vi "5.0.0_Task_Detect_Calibration.vi"(7 "Data in":T1, 8 "error in (no error)":errorcluster, 9 "AllControls In":T2, 10 "?":T3, 11 "Message Queue out":T4) -> (0 "error out":errorcluster, 1 "Flow":string, 2 "Data":T3, 3 "Message Queue Out":T4, 5 "Data out":T1)   [LabVIEW 2017]
uses:
  Depends/AMC/subVIs/TypeDefs/amc_Message Queue.ctl
  Depends/AMC/subVIs/TypeDefs/amc_Message.ctl
  Depends/Tools/Keyed Array/Tools_KeyedArray KeyedArray.ctl
  Ctrls/Data.ctl
  Ctrls/AllControls.ctl
  Ctrls/CSV_Data.ctl
  DIPC 692 Daemon API/typdef/calibration.ctl
  DIPC 692 Daemon API/typdef/task_detect_test_point.ctl
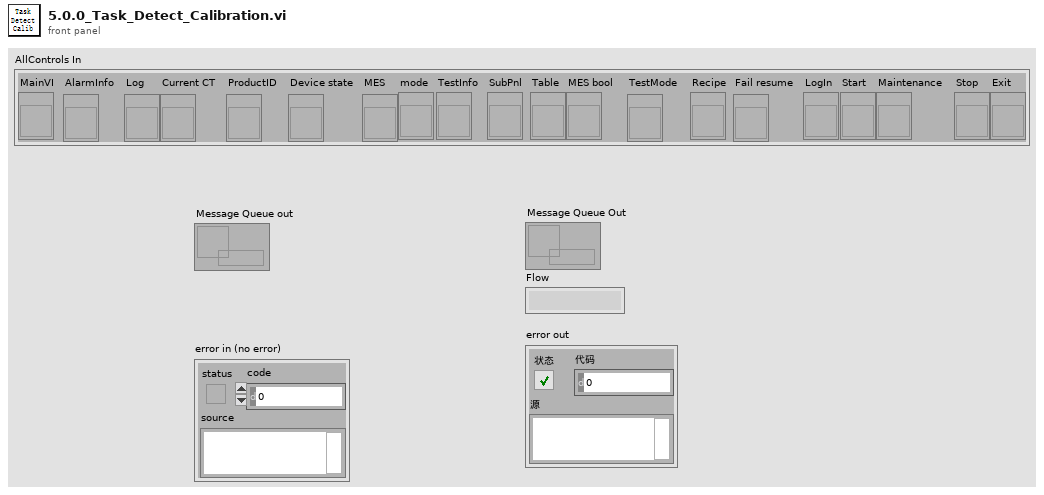
[diagram p1: front panel]
types:
  T1 = typedef "CSV_Data.ctl" = cluster{"Initialisation":cluster{"LMT - Connect UUT (con COM)":string, "LMT - Software Version (rrel)":string, "LMT - Write SKU file (wskuc)":string, "LMT - SKU file name":string, "Connect UUT DDM":string, "Read DDM EOL Timestamp - Mode":string, "Read DDM EOL Timestamp - Timestamp":string, "Read DDM EOL Timestamp - Rig ID":string, "Read DDM EOL Timestamp - Passmark ID":string, "Read DDM EOL Timestamp - Passmark Rev":string, "Software Version before flashing":string, "Read Hardware Serial":string, "UUT DDM SN":string, "Compare DDM SN with MES SN":string, "Backup PCBA Calibration EEPROM Response - CAL":string, "Flash Firmware Version":string, "Check SW Version":string, "Read DDM SW Version after flashing":string, "Set SKU Config":string, "Ready Status":string, "Set Device Mode to EOL":string, "DDM Parameter - Voltage":string, "DDM Parameter - Current":string, "DDM Parameter - Power":string, "DDM Parameter - Speed":string, "DDM Parameter - Pressure":string, "Tester Parameter - Voltage":string, "Tester Parameter - Current":string, "Tester Parameter - Power":string, "Tester Parameter - Ambient Pressure":string, "Tester Parameter - Ambient Temperature":string, "Calculated Parameter - DDM Pressure Corrected":string, "Calculated Parameter - DDM Real Power":string, "Calculated Parameter - Delta V":string}, "BEMF_Calibration":cluster{"Calibration Result - eol_cold_bemf_temp":string, "DDM Ambient Temp":string, "Restriction Plate Diameter":string, "Calibration Result - eol_bemf_mp_cold_coef_a":string, "Calibration Result - eol_bemf_mp_cold_coef_b":string, "Calibration Result - eol_bemf_mp_cold_coef_c":string, "Calibration Result - eol_bemf_lsi_cold_ref_coeffs":string, "Get - Calibration Result - eol_bemf_lsi_speed":string, "Get - Calibration Result - eol_bemf_lsi_integral_0":string, "Calibration Result - eol_bemf_lsi_integral_1":string, "Get - Calibration Result - eol_bemf_lsi_integral_2":string, "Get - Calibration Result - eol_cold_bemf":string, "Get - Calibration Result - eol_cold_bemf_fisf":string, "Finalise Calibration":string, "Compare -Calibration Result - eol_cold_bemf":string, "Compare -Calibration Result - eol_cold_bemf_fisf":string}, "ECO":cluster{"Reset Power Tune":string, "Reset BEMF FISF Calibration":string, "Restriction Plate Diameter":string, "ECO - Stabilisation Time":string, "ECO - DDM Parameter - Voltage":string, "ECO - DDM Parameter - Current":string, "ECO - DDM Parameter - Power":string, "ECO - DDM Parameter - Measured Power":string, "ECO - DDM Parameter - Speed":string, "ECO - DDM Parameter - Pressure":string, "ECO - Tester Parameter - Voltage":string, "ECO - Tester Parameter - Current":string, "ECO - Tester Parameter - Power":string, "ECO - Tester Parameter - Ambient Pressure":string, "ECO - Tester Parameter - Ambient Temperature":string, "ECO - Tester Parameter - Ambient Humidity":string, "ECO - Calculated Parameter - DDM Pressure Corrected":string, "ECO - Calculated Parameter - DDM Real Power":string, "ECO - Calculated Parameter - Delta V":string, "ECO - Calculated Parameter - Flowrate":string, "ECO - Calculated Parameter - Airwatt":string, "ECO - Formula":string, "PT ECO - Power Tune Mode Status":string}, "BOOST":cluster{"Restriction Plate Diameter":string, "BOOST - Stabilisation Time":string, "BOOST - DDM Parameter - Voltage":string, "BOOST - DDM Parameter - Current":string, "BOOST - DDM Parameter - Power":string, "BOOST - DDM Parameter - Measured Power":string, "BOOST - DDM Parameter - Speed":string, "BOOST - DDM Parameter - Pressure":string, "BOOST - Tester Parameter - Voltage":string, "BOOST - Tester Parameter - Current":string, "BOOST - Tester Parameter - Power":string, "BOOST - Tester Parameter - Ambient Pressure":string, "BOOST - Tester Parameter - Ambient Temperature":string, "BOOST - Tester Parameter - Ambient Humidity":string, "BOOST - Calculated Parameter - DDM Pressure Corrected":string, "BOOST - Calculated Parameter - DDM Real Power":string, "BOOST - Calculated Parameter - Delta V":string, "BOOST - Calculated Parameter - Flowrate":string, "BOOST - Calculated Parameter - Airwatt":string, "BOOST - Get AM Presence":string, "Air Muscle Turn Off Status":string, "BOOST - Air Muscle Calculated Parameter - Airwatt B":string, "BOOST - Air Muscle Calculate Airwatt Delta":string, "PT BOOST - Power Tune Mode Status":string, "Finalise Calibration":string, "ECO - Get AW Calibration value":string, "BOOST - Get AW Calibration value":string}, "MAX":cluster{"Restriction Plate Diameter":string, "MAX - Stabilisation Time":string, "Get Average Delta Tmag (LSIdelta_FISFdelta_LSItmag_FISFtmag_IIRtmag)":string, "Get Average Delta Tmag FISF":string, "MAX - DDM Parameter - Voltage":string, "MAX - DDM Parameter - Current":string, "MAX - DDM Parameter - Power":string, "MAX - DDM Parameter - Measured Power":string, "MAX - DDM Parameter - Speed":string, "MAX - DDM Parameter - Pressure":string, "MAX - Tester Parameter - Voltage":string, "MAX - Tester Parameter - Current":string, "MAX - Tester Parameter - Power":string, "MAX - Tester Parameter - Ambient Pressure":string, "MAX - Tester Parameter - Ambient Temperature":string, "MAX - Tester Parameter - Ambient Humidity":string, "MAX - Calculated Parameter - DDM Pressure Corrected":string, "MAX - Calculated Parameter - DDM Real Power":string, "MAX - Calculated Parameter - Delta V":string, "MAX - Calculated Parameter - Flowrate":string, "MAX - Calculated Parameter - Airwatt":string, "MAX_FISF_Check_Average_Delta_Tmag":string, "MAX - FISF - BEMF Finetune Result":string, "MAX tune - Delta P1":string, "MAX tune - Calculated Parameter - Airwatt":string, "Calculate Delta Airwatts - MAX finetune - Delta P2":string, "MAX finetune - DDM Parameter - Voltage":string, "MAX finetune - DDM Parameter - Current":string, "MAX finetune - DDM Parameter - Power":string, "MAX finetune - DDM Parameter - Measured Power":string, "MAX finetune - DDM Parameter - Speed":string, "MAX finetune - DDM Parameter - Pressure":string, "MAX finetune - Tester Parameter - Voltage":string, "MAX finetune - Tester Parameter - Current":string, "MAX finetune - Tester Parameter - Power":string, "MAX finetune - Tester Parameter - Ambient Pressure":string, "MAX finetune - Tester Parameter - Ambient Temperature":string, "MAX finetune - Tester Parameter - Ambient Humidity":string, "MAX finetune - Calculated Parameter - DDM Pressure Corrected":string, "MAX finetune - Calculated Parameter - DDM Real Power":string, "MAX finetune - Calculated Parameter - Delta V":string, "MAX finetune - Calculated Parameter - Flowrate":string, "MAX finetune - Calculated Parameter - Airwatt":string, "Check Derate Result":string, "Delta Tmag FISF":string, "Get Hot BEMF Result":string, "Calculate delta Pressure":string, "Finalise Calibration":string, "Calculate & Check Delta BEMF":string, "Delta P Airwatts Value":string}, "LL":cluster{"DDM Ambient Temp":string, "Restriction Plate Diameter":string, "LL - DDM Parameter - Voltage":string, "LL - DDM Parameter - Current":string, "LL - DDM Parameter - Power":string, "LL - DDM Parameter - Measured Power":string, "LL - DDM Parameter - Speed":string, "LL - DDM Parameter - Pressure":string, "LL - Tester Parameter - Voltage":string, "LL - Tester Parameter - Current":string, "LL - Tester Parameter - Power":string, "LL - DDM Real Power":string, "LL - Calibrate Task Detect LL":string}, "HL":cluster{"HL - DDM Parameter - Voltage":string, "HL - DDM Parameter - Current":string, "HL - DDM Parameter - Power":string, "HL - DDM Parameter - Measured Power":string, "HL - DDM Parameter - Speed":string, "HL - DDM Parameter - Pressure":string, "HL - Tester Parameter - Voltage":string, "HL - Tester Parameter - Current":string, "HL - Tester Parameter - Power":string, "HL - DDM Real Power":string, "HL - Calibrate Task Detect HL":string}, "LH":cluster{"Restriction Plate Diameter":string, "LH - DDM Parameter - Voltage":string, "LH - DDM Parameter - Current":string, "LH - DDM Parameter - Power":string, "LH - DDM Parameter - Measured Power":string, "LH - DDM Parameter - Speed":string, "LH - DDM Parameter - Pressure":string, "LH - Tester Parameter - Voltage":string, "LH - Tester Parameter - Current":string, "LH - Tester Parameter - Power":string, "LH - DDM Real Power":string, "LH - Calibrate Task Detect LH":string}, "HH":cluster{"HH - DDM Parameter - Voltage":string, "HH - DDM Parameter - Current":string, "HH - DDM Parameter - Power":string, "HH - DDM Parameter - Measured Power":string, "HH - DDM Parameter - Speed":string, "HH - DDM Parameter - Pressure":string, "HH - Tester Parameter - Voltage":string, "HH - Tester Parameter - Current":string, "HH - Tester Parameter - Power":string, "HH - DDM Real Power":string, "HH - Calibrate Task Detect HH":string}, "Inlet Blockage Calibration":cluster{"Inlet Blockage Calibration - DDM Parameter - Voltage":string, "Inlet Blockage Calibration - DDM Parameter - Current":string, "Inlet Blockage Calibration - DDM Parameter - Power":string, "Inlet Blockage Calibration - DDM Parameter - Measured Power":string, "Inlet Blockage Calibration - DDM Parameter - Speed":string, "Inlet Blockage Calibration - DDM Parameter - Pressure":string, "Inlet Blockage Calibration - Tester Parameter - Voltage":string, "Inlet Blockage Calibration - Tester Parameter - Current":string, "Inlet Blockage Calibration - Tester Parameter - Power":string, "Inlet Blockage Calibration - DDM Real Power":string, "Calibration Inlet Blockage_E":string, "Finalise Calibration":string, "Get Task Detect LL":string, "Get Task Detect HL":string, "Get Task Detect LH":string, "Get Task Detect HH":string, "Calibration Inlet Blockage":string, "Calibration eol cold bemf temp":string}, "GOOD":cluster{"GOOD UNIT - Clear EEPROM Error Log":string, "GOOD UNIT - Write Product Timestamp - Mode":string, "GOOD UNIT - Write Product Timestamp - Timestamp":string, "GOOD UNIT - Write Product Timestamp - Rig ID":string, "GOOD UNIT - Write Product Timestamp - Passmark ID":string, "GOOD UNIT - Write Product Timestamp - Passmark Rev":string, "GOOD UNIT - Set Device Mode to PROD":string, "GOOD UNIT - Backup PCBA Calibration EEPROM Response":string, "GOOD UNIT - Check Security Bit":string, "GOOD UNIT - Set Calibration Lock":string, "GOOD UNIT - Get_Calibration_Lock":string, "GOOD UNIT - Disconnect UUT":string}, "NG":cluster{"NG UNIT - Read NVM Error":string, "NG UNIT - Set Device Mode to FCT":string, "NG UNIT - Backup PCBA Calibration EEPROM Response - CAL":string, "NG UNIT - Backup PCBA Calibration EEPROM Response - ERROR":string, "NG UNIT - Backup PCBA Calibration EEPROM Response - USAGE":string, "NG UNIT - Disconnect UUT":string}, "SN":string, "Table":string[][], "Count":cluster{"Total":i32, "OK":i32, "NG":i32, "Yield":dbl}, "Start Time":timestamp, "daemon reference":refnum<k5>, "CT":dbl, "Config":string[][], "OK/NG":bool, "Station ID":string, "MES DDM SN":string, "MES PCBA SN":string, "Retest":string, "Lux":string, "Initialisation_Status":cluster{"LMT - Connect UUT (con COM)":string, "LMT - Software Version (rrel)":string, "LMT - Write SKU file (wskuc)":string, "LMT - SKU file name":string, "Connect UUT DDM":string, "Read DDM EOL Timestamp - Mode":string, "Read DDM EOL Timestamp - Timestamp":string, "Read DDM EOL Timestamp - Rig ID":string, "Read DDM EOL Timestamp - Passmark ID":string, "Read DDM EOL Timestamp - Passmark Rev":string, "Software Version before flashing":string, "Read Hardware Serial":string, "UUT DDM SN":string, "Compare DDM SN with MES SN":string, "Backup PCBA Calibration EEPROM Response - CAL":string, "Flash Firmware Version":string, "Check SW Version":string, "Read DDM SW Version after flashing":string, "Set SKU Config":string, "Ready Status":string, "Set Device Mode to EOL":string, "DDM Parameter - Voltage":string, "DDM Parameter - Current":string, "DDM Parameter - Power":string, "DDM Parameter - Speed":string, "DDM Parameter - Pressure":string, "Tester Parameter - Voltage":string, "Tester Parameter - Current":string, "Tester Parameter - Power":string, "Tester Parameter - Ambient Pressure":string, "Tester Parameter - Ambient Temperature":string, "Calculated Parameter - DDM Pressure Corrected":string, "Calculated Parameter - DDM Real Power":string, "Calculated Parameter - Delta V":string}, "BEMF_Calibration_Status":cluster{"Calibration Result - eol_cold_bemf_temp":string, "DDM Ambient Temp":string, "Restriction Plate Diameter":string, "Calibration Result - eol_bemf_mp_cold_coef_a":string, "Calibration Result - eol_bemf_mp_cold_coef_b":string, "Calibration Result - eol_bemf_mp_cold_coef_c":string, "Calibration Result - eol_bemf_lsi_cold_ref_coeffs":string, "Get - Calibration Result - eol_bemf_lsi_speed":string, "Get - Calibration Result - eol_bemf_lsi_integral_0":string, "Calibration Result - eol_bemf_lsi_integral_1":string, "Get - Calibration Result - eol_bemf_lsi_integral_2":string, "Get - Calibration Result - eol_cold_bemf":string, "Get - Calibration Result - eol_cold_bemf_fisf":string, "Finalise Calibration":string, "Compare -Calibration Result - eol_cold_bemf":string, "Compare -Calibration Result - eol_cold_bemf_fisf":string}, "ECO_Status":cluster{"Reset Power Tune":string, "Reset BEMF FISF Calibration":string, "Restriction Plate Diameter":string, "ECO - Stabilisation Time":string, "ECO - DDM Parameter - Voltage":string, "ECO - DDM Parameter - Current":string, "ECO - DDM Parameter - Power":string, "ECO - DDM Parameter - Measured Power":string, "ECO - DDM Parameter - Speed":string, "ECO - DDM Parameter - Pressure":string, "ECO - Tester Parameter - Voltage":string, "ECO - Tester Parameter - Current":string, "ECO - Tester Parameter - Power":string, "ECO - Tester Parameter - Ambient Pressure":string, "ECO - Tester Parameter - Ambient Temperature":string, "ECO - Tester Parameter - Ambient Humidity":string, "ECO - Calculated Parameter - DDM Pressure Corrected":string, "ECO - Calculated Parameter - DDM Real Power":string, "ECO - Calculated Parameter - Delta V":string, "ECO - Calculated Parameter - Flowrate":string, "ECO - Calculated Parameter - Airwatt":string, "ECO - Formula":string, "PT ECO - Power Tune Mode Status":string}, "BOOST_Status":cluster{"Restriction Plate Diameter":string, "BOOST - Stabilisation Time":string, "BOOST - DDM Parameter - Voltage":string, "BOOST - DDM Parameter - Current":string, "BOOST - DDM Parameter - Power":string, "BOOST - DDM Parameter - Measured Power":string, "BOOST - DDM Parameter - Speed":string, "BOOST - DDM Parameter - Pressure":string, "BOOST - Tester Parameter - Voltage":string, "BOOST - Tester Parameter - Current":string, "BOOST - Tester Parameter - Power":string, "BOOST - Tester Parameter - Ambient Pressure":string, "BOOST - Tester Parameter - Ambient Temperature":string, "BOOST - Tester Parameter - Ambient Humidity":string, "BOOST - Calculated Parameter - DDM Pressure Corrected":string, "BOOST - Calculated Parameter - DDM Real Power":string, "BOOST - Calculated Parameter - Delta V":string, "BOOST - Calculated Parameter - Flowrate":string, "BOOST - Calculated Parameter - Airwatt":string, "BOOST - Get AM Presence":string, "Air Muscle Turn Off Status":string, "BOOST - Air Muscle Calculated Parameter - Airwatt B":string, "BOOST - Air Muscle Calculate Airwatt Delta":string, "PT BOOST - Power Tune Mode Status":string, "Finalise Calibration":string, "ECO - Get AW Calibration value":string, "BOOST - Get AW Calibration value":string}, "MAX_Status":cluster{"Restriction Plate Diameter":string, "MAX - Stabilisation Time":string, "Get Average Delta Tmag (LSIdelta_FISFdelta_LSItmag_FISFtmag_IIRtmag)":string, "Get Average Delta Tmag FISF":string, "MAX - DDM Parameter - Voltage":string, "MAX - DDM Parameter - Current":string, "MAX - DDM Parameter - Power":string, "MAX - DDM Parameter - Measured Power":string, "MAX - DDM Parameter - Speed":string, "MAX - DDM Parameter - Pressure":string, "MAX - Tester Parameter - Voltage":string, "MAX - Tester Parameter - Current":string, "MAX - Tester Parameter - Power":string, "MAX - Tester Parameter - Ambient Pressure":string, "MAX - Tester Parameter - Ambient Temperature":string, "MAX - Tester Parameter - Ambient Humidity":string, "MAX - Calculated Parameter - DDM Pressure Corrected":string, "MAX - Calculated Parameter - DDM Real Power":string, "MAX - Calculated Parameter - Delta V":string, "MAX - Calculated Parameter - Flowrate":string, "MAX - Calculated Parameter - Airwatt":string, "MAX_FISF_Check_Average_Delta_Tmag":string, "MAX - FISF - BEMF Finetune Result":string, "MAX tune - Delta P1":string, "MAX tune - Calculated Parameter - Airwatt":string, "Calculate Delta Airwatts - MAX finetune - Delta P2":string, "MAX finetune - DDM Parameter - Voltage":string, "MAX finetune - DDM Parameter - Current":string, "MAX finetune - DDM Parameter - Power":string, "MAX finetune - DDM Parameter - Measured Power":string, "MAX finetune - DDM Parameter - Speed":string, "MAX finetune - DDM Parameter - Pressure":string, "MAX finetune - Tester Parameter - Voltage":string, "MAX finetune - Tester Parameter - Current":string, "MAX finetune - Tester Parameter - Power":string, "MAX finetune - Tester Parameter - Ambient Pressure":string, "MAX finetune - Tester Parameter - Ambient Temperature":string, "MAX finetune - Tester Parameter - Ambient Humidity":string, "MAX finetune - Calculated Parameter - DDM Pressure Corrected":string, "MAX finetune - Calculated Parameter - DDM Real Power":string, "MAX finetune - Calculated Parameter - Delta V":string, "MAX finetune - Calculated Parameter - Flowrate":string, "MAX finetune - Calculated Parameter - Airwatt":string, "Check Derate Result":string, "Delta Tmag FISF":string, "Get Hot BEMF Result":string, "Calculate delta Pressure":string, "Finalise Calibration":string, "Calculate & Check Delta BEMF":string, "Delta P Airwatts Value":string}, "LL_Status":cluster{"DDM Ambient Temp":string, "Restriction Plate Diameter":string, "LL - DDM Parameter - Voltage":string, "LL - DDM Parameter - Current":string, "LL - DDM Parameter - Power":string, "LL - DDM Parameter - Measured Power":string, "LL - DDM Parameter - Speed":string, "LL - DDM Parameter - Pressure":string, "LL - Tester Parameter - Voltage":string, "LL - Tester Parameter - Current":string, "LL - Tester Parameter - Power":string, "LL - DDM Real Power":string, "LL - Calibrate Task Detect LL":string}, "HL_Status":cluster{"HL - DDM Parameter - Voltage":string, "HL - DDM Parameter - Current":string, "HL - DDM Parameter - Power":string, "HL - DDM Parameter - Measured Power":string, "HL - DDM Parameter - Speed":string, "HL - DDM Parameter - Pressure":string, "HL - Tester Parameter - Voltage":string, "HL - Tester Parameter - Current":string, "HL - Tester Parameter - Power":string, "HL - DDM Real Power":string, "HL - Calibrate Task Detect HL":string}, "LH_Status":cluster{"Restriction Plate Diameter":string, "LH - DDM Parameter - Voltage":string, "LH - DDM Parameter - Current":string, "LH - DDM Parameter - Power":string, "LH - DDM Parameter - Measured Power":string, "LH - DDM Parameter - Speed":string, "LH - DDM Parameter - Pressure":string, "LH - Tester Parameter - Voltage":string, "LH - Tester Parameter - Current":string, "LH - Tester Parameter - Power":string, "LH - DDM Real Power":string, "LH - Calibrate Task Detect LH":string}, "HH_Status":cluster{"HH - DDM Parameter - Voltage":string, "HH - DDM Parameter - Current":string, "HH - DDM Parameter - Power":string, "HH - DDM Parameter - Measured Power":string, "HH - DDM Parameter - Speed":string, "HH - DDM Parameter - Pressure":string, "HH - Tester Parameter - Voltage":string, "HH - Tester Parameter - Current":string, "HH - Tester Parameter - Power":string, "HH - DDM Real Power":string, "HH - Calibrate Task Detect HH":string}, "Inlet Blockage Calibration_Status":cluster{"Inlet Blockage Calibration - DDM Parameter - Voltage":string, "Inlet Blockage Calibration - DDM Parameter - Current":string, "Inlet Blockage Calibration - DDM Parameter - Power":string, "Inlet Blockage Calibration - DDM Parameter - Measured Power":string, "Inlet Blockage Calibration - DDM Parameter - Speed":string, "Inlet Blockage Calibration - DDM Parameter - Pressure":string, "Inlet Blockage Calibration - Tester Parameter - Voltage":string, "Inlet Blockage Calibration - Tester Parameter - Current":string, "Inlet Blockage Calibration - Tester Parameter - Power":string, "Inlet Blockage Calibration - DDM Real Power":string, "Calibration Inlet Blockage_E":string, "Finalise Calibration":string, "Get Task Detect LL":string, "Get Task Detect HL":string, "Get Task Detect LH":string, "Get Task Detect HH":string, "Calibration Inlet Blockage":string, "Calibration eol cold bemf temp":string}, "GOOD_Status":cluster{"GOOD UNIT - Clear EEPROM Error Log":string, "GOOD UNIT - Write Product Timestamp - Mode":string, "GOOD UNIT - Write Product Timestamp - Timestamp":string, "GOOD UNIT - Write Product Timestamp - Rig ID":string, "GOOD UNIT - Write Product Timestamp - Passmark ID":string, "GOOD UNIT - Write Product Timestamp - Passmark Rev":string, "GOOD UNIT - Set Device Mode to PROD":string, "GOOD UNIT - Backup PCBA Calibration EEPROM Response":string, "GOOD UNIT - Check Security Bit":string, "GOOD UNIT - Set Calibration Lock":string, "GOOD UNIT - Get_Calibration_Lock":string, "GOOD UNIT - Disconnect UUT":string}, "NG_Status":cluster{"NG UNIT - Read NVM Error":string, "NG UNIT - Set Device Mode to FCT":string, "NG UNIT - Backup PCBA Calibration EEPROM Response - CAL":string, "NG UNIT - Backup PCBA Calibration EEPROM Response - ERROR":string, "NG UNIT - Backup PCBA Calibration EEPROM Response - USAGE":string, "NG UNIT - Disconnect UUT":string}, "SKU":string, "Plate_Diameter":string, "Alarm":string}
  T2 = typedef "AllControls.ctl" = cluster{"MainVI":refnum<vi>, "AlarmInfo":refnum<vi>, "Log":refnum<vi>, "Current CT":refnum<vi>, "ProductID":refnum<vi>, "Device state":refnum<vi>, "MES":refnum<vi>, "mode":refnum<vi>, "TestInfo":refnum<vi>, "SubPnl":refnum<vi>, "Table":refnum<vi>, "MES bool":refnum<vi>, "TestMode":refnum<vi>, "Recipe":refnum<vi>, "Fail resume":refnum<vi>, "LogIn":refnum<vi>, "Start":refnum<vi>, "Maintenance":refnum<vi>, "Stop":refnum<vi>, "Exit":refnum<vi>}
  T3 = typedef "Data.ctl" = cluster{"Initialisation":cluster{"DDM_Parameter":dbl[], "DDM_Parameter_status":bool[], "Get_Tester_Parameter":dbl[], "Get_Tester_Parameter_status":bool[], "Cal_Tester_Parameter":dbl[], "Cal_Tester_Parameter_status":bool[], "sw_version_before_status":bool, "sw_version_after_status":bool, "Set_SKU_Config_With_LMT_status":bool, "FCT_timestamp_status":bool, "LMT_Connect_to_UUT_status":bool}, "BEMF_Calibration":cluster{"Read_ambient_temperature":dbl, "Calibration_Vaule":dbl[], "Calibration_Vaule _B":dbl[], "Calibration_Vaule_status":bool[], "Calibration_Vaule_B_status":bool[]}, "ECO":cluster{"DDM_Parameter":dbl[], "DDM_Parameter_status":bool[], "Get_Tester_Parameter":dbl[], "Get_Tester_Parameter_status":bool[], "Cal_Tester_Parameter":dbl[], "Cal_Tester_Parameter_status":bool[], "DDM_Parameter_after_power_tune":dbl[], "Get_Tester_Parameter_after_power_tune":dbl[], "Cal_Tester_Parameter_after_power_tune":dbl[], "Cal_Tester_Parameter_after_power_tune_status":bool[], "Delta_P":dbl}, "BOOST":cluster{"DDM_Parameter":dbl[], "DDM_Parameter_status":bool[], "Get_Tester_Parameter":dbl[], "Get_Tester_Parameter_status":bool[], "Cal_Tester_Parameter":dbl[], "Cal_Tester_Parameter_status":bool[], "DDM_Parameter_after_power_tune":dbl[], "Get_Tester_Parameter_after_power_tune":dbl[], "Cal_Tester_Parameter_after_power_tune":dbl[], "Cal_Tester_Parameter_after_power_tune_status":bool[], "airwatts_am_off":dbl, "AW_Delta_(AM_on_and_off)":dbl, "AW_Delta_(AM_on_and_off)_Status":bool, "Delta_P":dbl}, "MAX":cluster{"Average_Tmag_Data":cluster{"LSI Delta in degC":dbl, "FISF Delta in degc":dbl, "LSI Tmag in degC":dbl, "Fisf Tmag in degC":dbl, "IIR Tmag in degC":dbl}, "DDM_Parameter":dbl[], "DDM_Parameter_status":bool[], "Get_Tester_Parameter":dbl[], "Get_Tester_Parameter_status":bool[], "Cal_Tester_Parameter":dbl[], "BEMF_Finetune":cluster{"eol_bemf_mp_cold_coef_c":dbl, "eol_cold_bemf_fisf_offset":dbl}, "AW_Tune":cluster{"delta_P1":dbl, "delta_P_Setting":dbl}, "DDM_Parameter_after_Airwatts_Tune":dbl[], "Get_Tester_Parameter_after_Airwatts_Tune":dbl[], "Cal_Tester_Parameter_after_Airwatts_Tune":dbl[], "DDM_Parameter_after_Airwatts_Finetune":dbl[], "Get_Tester_Parameter_after_Airwatts_Finetune":dbl[], "Cal_Tester_Parameter_after_Airwatts_Finetune":dbl[], "AW_Finetune":cluster{"delta_P2":dbl, "delta_P_Setting":dbl}, "Delta_Tmag_after_tune":cluster{"LSI Delta in degC":dbl, "FISF Delta in degc":dbl, "LSI Tmag in degC":dbl, "Fisf Tmag in degC":dbl, "IIR Tmag in degC":dbl}, "Hot Bemf in mV":dbl, "DDM_Pressure":dbl, "Delta_Pressure":dbl, " Cold Bemf in mV":dbl, " delta Bemf":dbl, " delta p":dbl, "Delta_Pressure_status":bool, " delta Bemf_status":bool, "LSI Delta in degC_status":bool, "FISF Delta in degc_status":bool, "Max_check_derate_status_status":bool, "Average_All_data":dbl[][], "Average_Tmag_Data_status":bool[], "Average_Tmag_Data_after_tune_status":bool[], "Cal_Tester_Parameter_status":bool[], "Cal_Tester_Parameter_status_after_Airwatts_Tune":bool[], "Cal_Tester_Parameter_status_after_Airwatts_FineTune":bool[]}, "Task_Detect_Calib":cluster{"LL":cluster{"DDM_Parameter":dbl[], "DDM_Parameter_status":bool[], "Get_Tester_Parameter":dbl[], "Get_Tester_Parameter_status":bool[], "Set_task_detect_A":dbl, "Set_task_detect_A_Status":bool}, "HL":cluster{"DDM_Parameter":dbl[], "DDM_Parameter_status":bool[], "Get_Tester_Parameter":dbl[], "Get_Tester_Parameter_status":bool[], "Set_task_detect_B":dbl, "Set_task_detect_B_Status":bool}, "LH":cluster{"DDM_Parameter":dbl[], "DDM_Parameter_status":bool[], "Get_Tester_Parameter":dbl[], "Get_Tester_Parameter_status":bool[], "Set_task_detect_C":dbl, "Set_task_detect_C_Status":bool}, "HH":cluster{"DDM_Parameter":dbl[], "DDM_Parameter_status":bool[], "Get_Tester_Parameter":dbl[], "Get_Tester_Parameter_status":bool[], "Set_task_detect_D":dbl, "Read_and_check_calibration_Status":bool[], "Set_task_detect_D_Status":bool}, "Get_eol_inlet_blockage_E":dbl, "Calib_vaule":cluster{"Get_task_detect_LL":dbl, "Get_task_detect_HL":dbl, "Get_task_detect_LH":dbl, "Get_task_detect_HH":dbl, "eol_inlet_blockage":dbl, "eol_code_bemf_temp":dbl}, "calibrated temp":dbl, "Inlet_Blockage_Calibration":cluster{"DDM_Parameter":dbl[], "DDM_Parameter_status":bool[], "Get_Tester_Parameter":dbl[], "Get_Tester_Parameter_status":bool[]}, "Get_eol_inlet_blockage_E_Status":bool}, "good":cluster{"Write_Product_TS":cluster{"TIMESTAMP":i64, "RIG_ID":i64, "PASSMARK_ID":i64, "PASSMARK_REV":i64}, "Read_Product_TS":cluster{"TIMESTAMP":i64, "RIG_ID":i64, "PASSMARK_ID":i64, "PASSMARK_REV":i64}, "Good_Check_Secuity_Bit_Stauts":bool}}
  T4 = typedef "amc_Message Queue.ctl" = refnum<queue>
  T5 = typedef "HD Config.ctl" = cluster{" PC":cluster{"PC Address":u8[], "PC Port":i32}, "FCO":cluster{"COM":refnum<visa-resource-name>, "Baudrate":u32}, "DC Power ":cluster{"COM":refnum<visa-resource-name>, "Baudrate":u32}, "PW3336":cluster{"COM":refnum<visa-resource-name>, "Baudrate":u32}, "Lefoo":cluster{"COM":refnum<visa-resource-name>, "Baudrate":u32}, "Tempt&Hum":cluster{"COM":refnum<visa-resource-name>, "Baudrate":u32}, "DIPC":cluster{"COM":refnum<visa-resource-name>}, "Daemon":cluster{"IP Address":string, "Port":u16, "Retry":u16}, "URAT":cluster{"COM":refnum<visa-resource-name>, "Baudrate":u32}, "Fail_resume_mode":bool, "GRR":bool}
  T6 = typedef "calibration.ctl" = string
  T7 = typedef "task_detect_test_point.ctl" = enum16{"LL", "HL", "LH", "HH"}
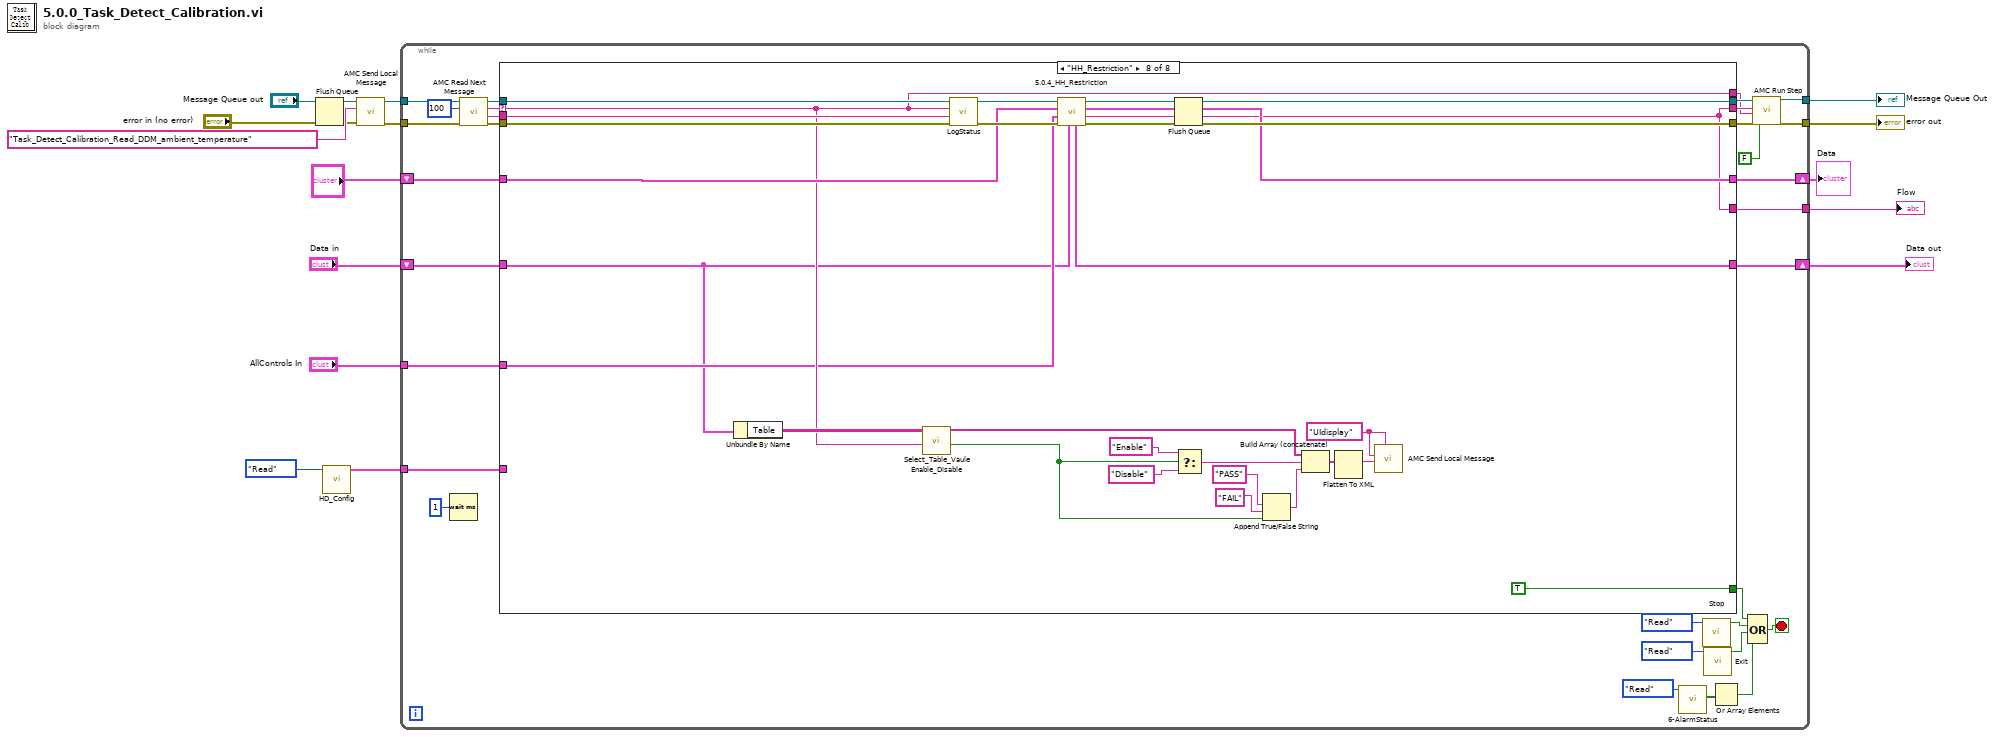
[diagram p0: block diagram]
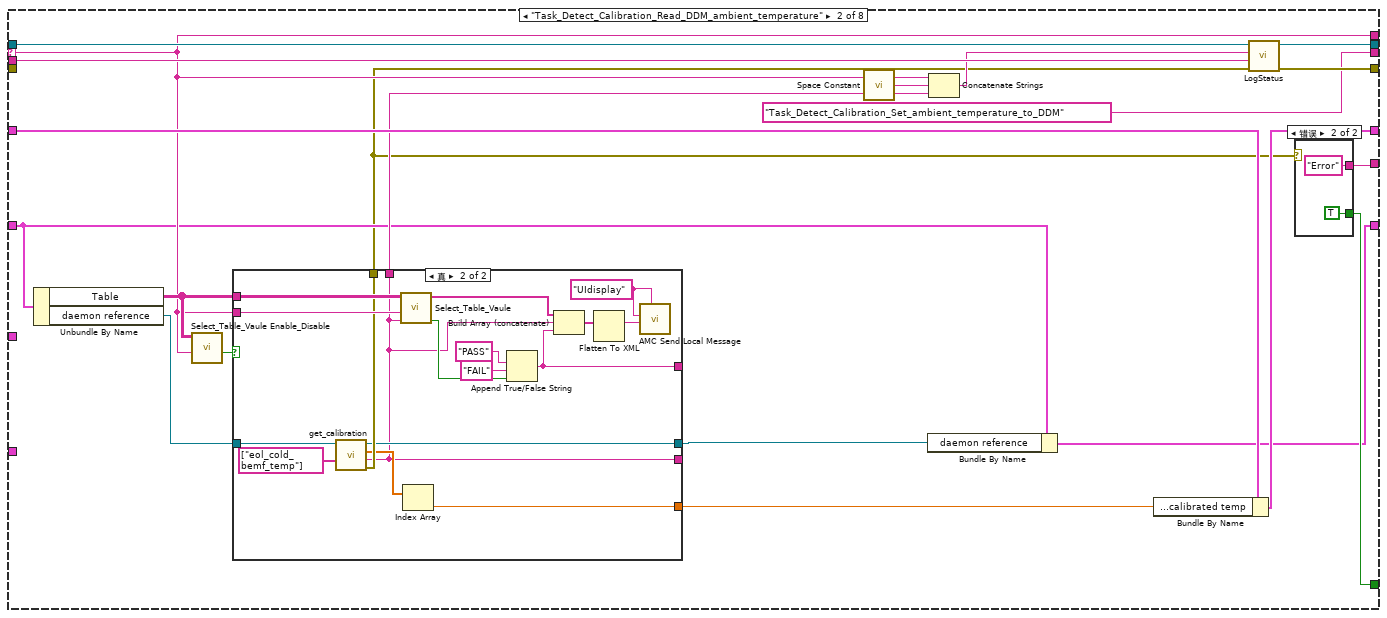
[diagram p3: hidden frame]
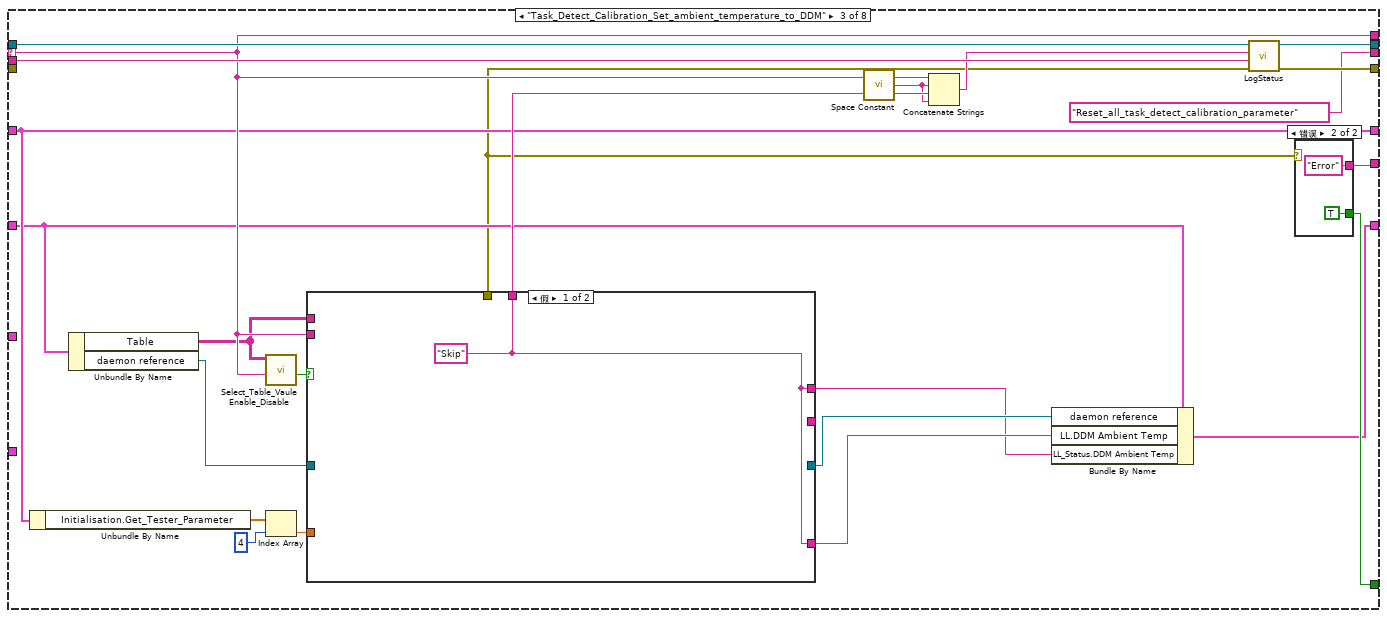
[diagram p6: hidden frame]
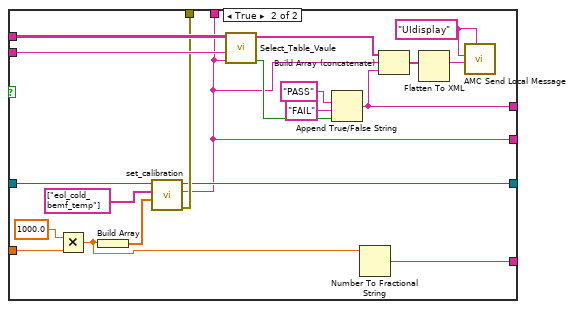
[diagram p8: hidden frame]
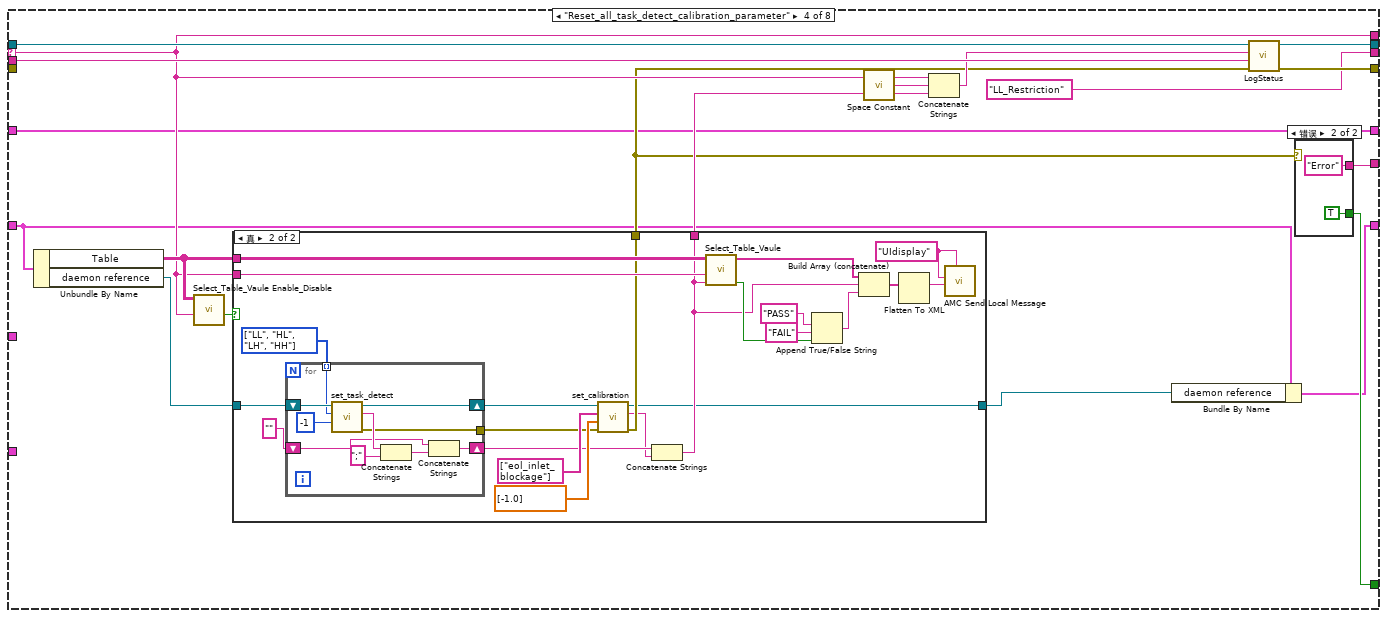
[diagram p9: hidden frame]
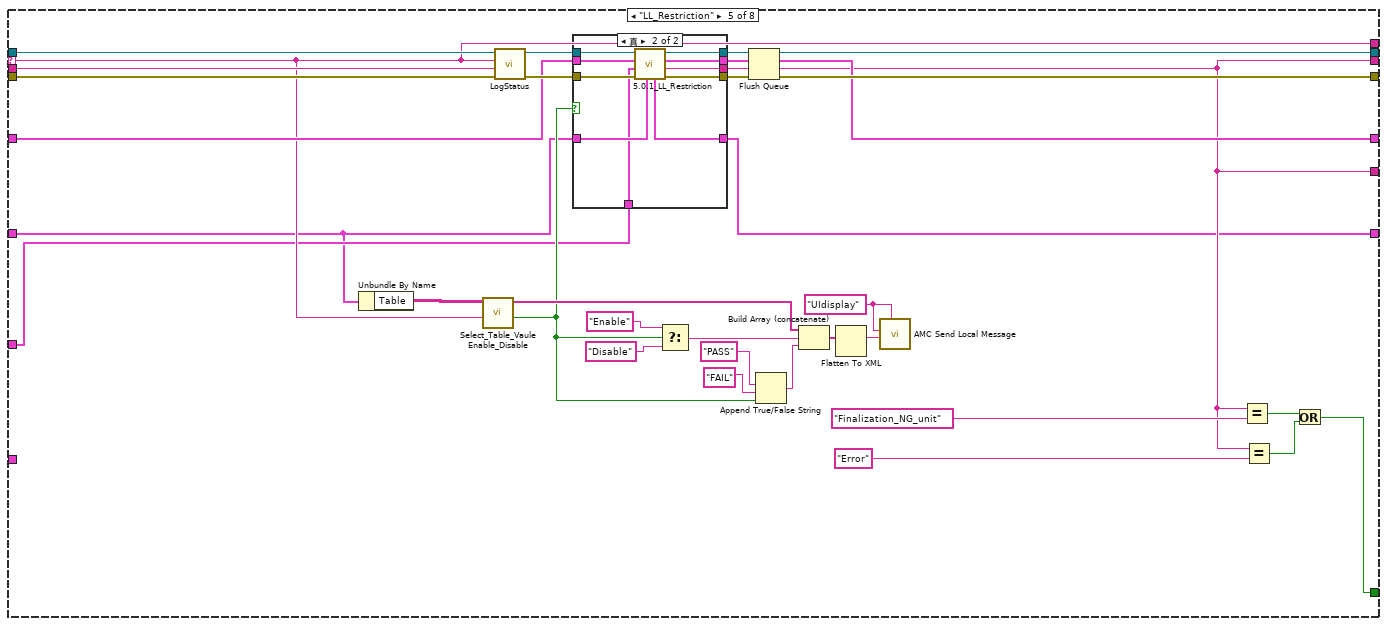
[diagram p12: hidden frame]
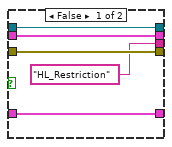
[diagram p13: hidden frame]
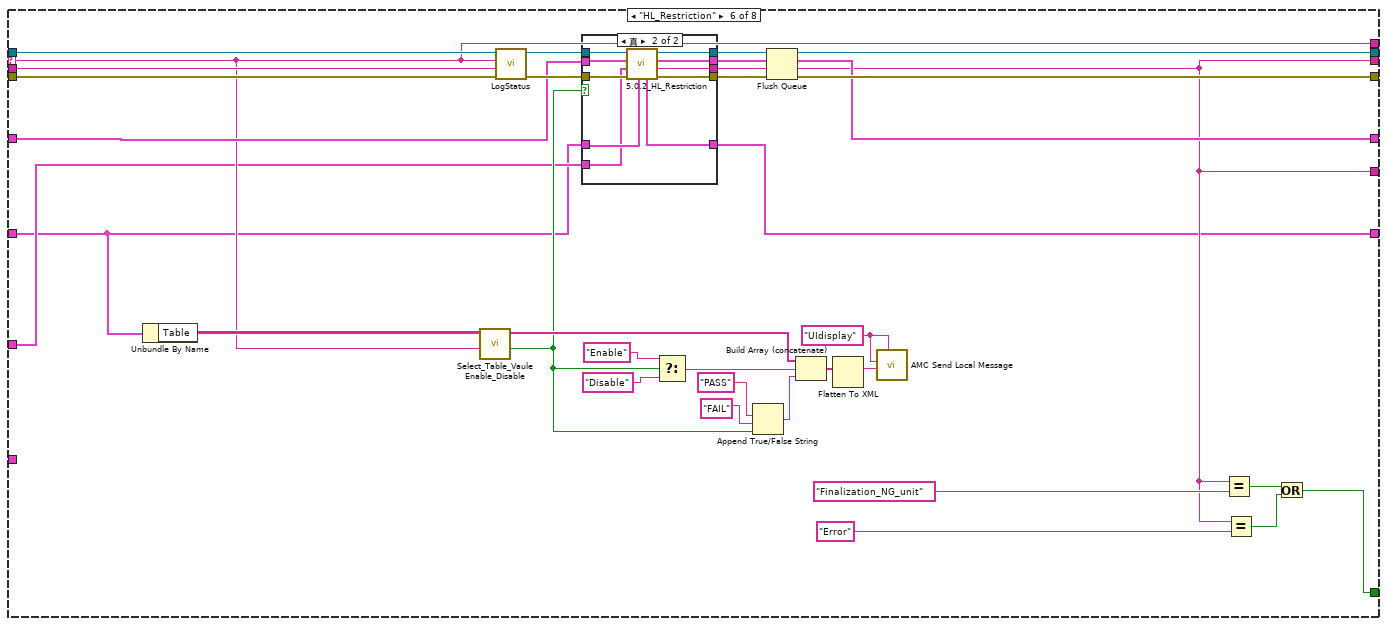
[diagram p14: hidden frame]
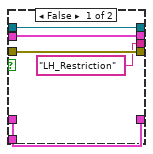
[diagram p15: hidden frame]
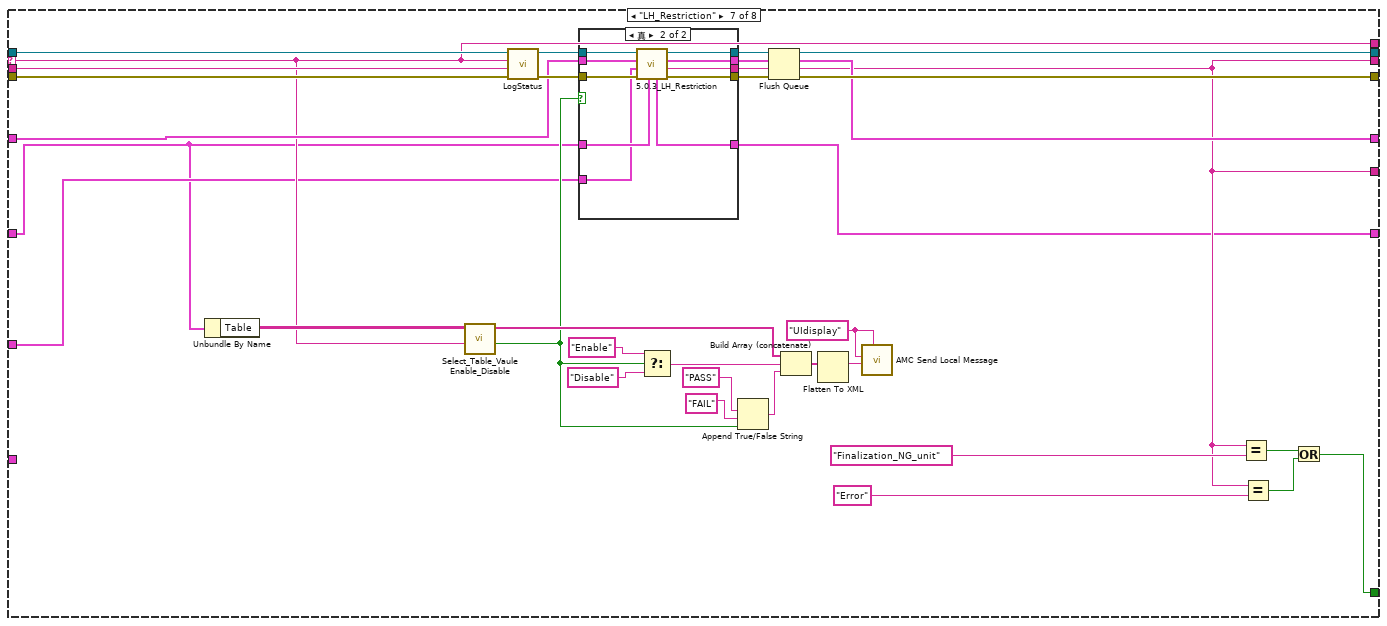
[diagram p16: hidden frame]
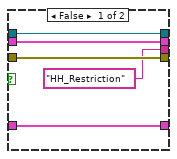
[diagram p17: hidden frame]
diagram:
  n1 = Flush Queue(queue="Message Queue out") -> (queue out=w4:T4)  [unwired: 1 in, 2 out]
  n2 = call "HD_Config.vi"("Step"=enum16{"Initial", "Write", "Read"}."Read") -> ("HD Config out"=w8:T5)  [unwired: 9 in, 1 out]
  n3 = call "AMC Send Local Message.vi"("error in (no error)"="error in (no error)", "Message Name"="Task_Detect_Calibration_Read_DDM_ambient_temperature", "Message Queue in"=w4) -> ("error out"=w13:errorcluster, "Message Queue out"=w14:T4)  [unwired: 7 in]
  n4 = while {
    tunnel: w14 -> [w47]
    tunnel: [w43] -> w6
    tunnel: w13 -> [w41]
    tunnel: [w38] -> w5
    shift-right: [w34] -> w10
    shift-left: "?" -> [w35]
    tunnel: w8 -> [w33]
    tunnel: [w29] -> w7
    shift-right: [w21] -> w2
    shift-left: "Data in" -> [w22]
    tunnel: "AllControls In" -> [w20]
    stop <- w23 stop-if-true
    n5 = Wait (ms)(milliseconds to wait=u32 1 ("等待时间（毫秒）")) -> ()  [unwired: 1 out]
    n6 = call "AMC Read Next Message.vi"("error in (no error)"=w41, "timeout (1ms)"=100, "Message Queue in"=w47) -> ("error out"=w40:errorcluster, "Message Value"=w31:string, "Message Name"=w45:string, "Message Queue out"=w46:T4)  [unwired: 1 in, 4 out]
    n7 = case shown="\"HH_Restriction\"" w45 {
      selector: w45 -> [_ w62 w108 w147 w197 w241 w287 w333]
      tunnel: w46 -> [w51 w71 w114 w155 w217 w263 w309 w351]
      tunnel: [w51 w71 w114 w155 w201 w253 w299 w345] -> w44
      tunnel: w40 -> [w50 _ _ _ w221 w267 w313 w355]
      tunnel: [w50 w70 w113 w154 w218 w264 w310 w352] -> w39
      tunnel: [_ w58 w105 w143 w206 w254 w301 TRUE] -> w24
      tunnel: w35 -> [w49 w67 w99 w141 w208 w260 w306 w348]
      tunnel: [w49 w56 w99 w141 w215 w261 w307 w349] -> w34
      tunnel: w31 -> [_ w69 w112 w153 w220 w266 w312 w354]
      tunnel: [_ w62 w108 w147 w197 w241 w287 w333] -> w30
      tunnel: w33 -> [_ _ _ _ _ _ _ _]
      tunnel: [_ "Task_Detect_Calibration_Set_ambient_temperature_to_DDM" "Reset_all_task_detect_calibration_parameter" "LL_Restriction" w202 w255 w300 w347] -> w32
      tunnel: [_ w59 w106 w144 w202 w255 w300 w347] -> w29
      tunnel: w22 -> [w48 w55 w98 w140 w191 w237 w283 w329]
      tunnel: [w48 w53 w97 w139 w193 w239 w285 w330] -> w21
      tunnel: w20 -> [_ _ _ _ w192 w238 w284 w331]
      frame "假", Default {
      }
      frame "Task_Detect_Calibration_Read_DDM_ambient_temperature" {
        n8 = Unbundle By Name(w55) -> ("Table"=w63:string[][], "daemon reference"=w60:refnum<k5>)
        n9 = call "Select_Table_Vaule Enable_Disable.vi"("Action"=w62, "Table"=w63) -> ("Enable"=w61:bool)  [unwired: 8 in, 1 out]
        n10 = case shown="真" w61 {
          tunnel: [_ w76] -> w64
          tunnel: w63 -> [_ w84]
          tunnel: w62 -> [_ w83]
          tunnel: w60 -> [w74 w81]
          tunnel: [_ w80] -> w54
          tunnel: [w74 w78] -> w52
          tunnel: [_ w77] -> w57
          tunnel: [_ w76] -> _
          tunnel: [_ w75] -> _
          frame False {
          }
          frame True {
            w90 = "UIdisplay" ("Process (\"\" - local)")
            n11 = call "get_calibration.vi"("Calibration"=T6[] ["eol_cold_bemf_temp"], "daemon reference in"=w81) -> ("error out"=w80:errorcluster, "response"=w76:string, "values"=w79:dbl[], "daemon reference out"=w78:refnum<k5>)  [unwired: 5 in, 1 out]
            n12 = call "Select_Table_Vaule.vi"("Vaule"=w76, "Action"=w83, "Table"=w84) -> ("Result"=w85:bool, "vaule"=w91:string[])  [unwired: 7 in]
            n13 = Index Array(array=w79) -> (element=w77:dbl)  [unwired: 1 in]
            n14 = Append True/False String(1:w85, 2:"FAIL" ("真字符串"), 3:"PASS" ("真字符串")) -> (0:w75:string)  [unwired: 1 in]
            n15 = Build Array (concatenate)(w91, w76, w75) -> (w89:string[])
            n16 = Flatten To XML(anything=w89) -> (xml string=w88:string)
            n17 = call "AMC Send Local Message.vi"("Process (\"\" - local)"=w90, "Message Value"=w88, "Message Name"=w90) -> ()  [unwired: 7 in, 2 out]
          }
        }
        n18 = call <vilib>:"Space Constant.vi"() -> ("String"=w65:string)
        n19 = Bundle By Name(cluster=w55, "daemon reference"=w52) -> (w53:T1)
        n20 = Concatenate Strings(w62, w65, w64) -> (w66:string)
        n21 = Bundle By Name(cluster=w67, "Task_Detect_Calib.calibrated temp"=w57) -> (w56:T3)
        n22 = call "LogStatus.vi"("error in (no error)"=w54, "last message"=w69, "message"=w66) -> ("error  out"=w70:errorcluster)  [unwired: 8 in]
        n23 = case shown="错误" w54 {
          tunnel: [_ TRUE] -> w58
          tunnel: [_ "Error"] -> w59
          frame No Error {
          }
          frame Error {
          }
        }
      }
      frame "Task_Detect_Calibration_Set_ambient_temperature_to_DDM" {
        n24 = Unbundle By Name(w99) -> ("Initialisation.Get_Tester_Parameter"=w104:dbl[])
        n25 = Unbundle By Name(w98) -> ("Table"=w101:string[][], "daemon reference"=w100:refnum<k5>)
        n26 = call "Select_Table_Vaule Enable_Disable.vi"("Action"=w108, "Table"=w101) -> ("Enable"=w107:bool)  [unwired: 8 in, 1 out]
        n27 = Index Array(array=w104, index=4) -> (element=w103:dbl)
        n28 = case shown="假" w107 {
          tunnel: [w117 w121] -> w109
          tunnel: w101 -> [_ w130]
          tunnel: w108 -> [_ w129]
          tunnel: w100 -> [_ w126]
          tunnel: [_ w127] -> w95
          tunnel: w103 -> [_ w125]
          tunnel: [_ w122] -> w96
          tunnel: [_ w121] -> _
          tunnel: [w117 w120] -> w92
          tunnel: [w117 w118] -> w93
          frame False {
            w117 = "Skip" ("response")
          }
          frame True {
            w136 = "UIdisplay" ("Process (\"\" - local)")
            n29 = Multiply(x=1000.0, y=w125) -> (x*y=w119:dbl)
            n30 = Build Array(w119) -> (w124:dbl[])
            n31 = call "set_calibration.vi"("values"=w124, "calibration"=T6[] ["eol_cold_bemf_temp"], "daemon reference in"=w126) -> ("error out"=w127:errorcluster, "response"=w121:string, "daemon reference out"=w122:refnum<k5>)  [unwired: 5 in, 1 out]
            n32 = call "Select_Table_Vaule.vi"("Vaule"=w121, "Action"=w129, "Table"=w130) -> ("Result"=w131:bool, "vaule"=w137:string[])  [unwired: 7 in]
            n33 = Append True/False String(1:w131, 2:"FAIL" ("真字符串"), 3:"PASS" ("真字符串")) -> (0:w120:string)  [unwired: 1 in]
            n34 = Number To Fractional String(number=w119) -> (F-format string=w118:string)  [unwired: 3 in]
            n35 = Build Array (concatenate)(w137, w121, w120) -> (w135:string[])
            n36 = Flatten To XML(anything=w135) -> (xml string=w134:string)
            n37 = call "AMC Send Local Message.vi"("Process (\"\" - local)"=w136, "Message Value"=w134, "Message Name"=w136) -> ()  [unwired: 7 in, 2 out]
          }
        }
        n38 = call <vilib>:"Space Constant.vi"() -> ("String"=w94:string)
        n39 = Concatenate Strings(w108, w94, w109, w94) -> (w110:string)
        n40 = Bundle By Name(cluster=w98, "daemon reference"=w96, "LL.DDM Ambient Temp"=w93, "LL_Status.DDM Ambient Temp"=w92) -> (w97:T1)
        n41 = call "LogStatus.vi"("error in (no error)"=w95, "last message"=w112, "message"=w110) -> ("error  out"=w113:errorcluster)  [unwired: 8 in]
        n42 = case shown="错误" w95 {
          tunnel: [_ TRUE] -> w105
          tunnel: [_ "Error"] -> w106
          frame No Error {
          }
          frame Error {
          }
        }
      }
      frame "Reset_all_task_detect_calibration_parameter" {
        n43 = Unbundle By Name(w140) -> ("Table"=w148:string[][], "daemon reference"=w145:refnum<k5>)
        n44 = call "Select_Table_Vaule Enable_Disable.vi"("Action"=w147, "Table"=w148) -> ("Enable"=w146:bool)  [unwired: 8 in, 1 out]
        n45 = case shown="真" w146 {
          tunnel: [_ w163] -> w149
          tunnel: w148 -> [_ w172]
          tunnel: w147 -> [_ w171]
          tunnel: w145 -> [w158 w170]
          tunnel: [_ w161] -> w142
          tunnel: [w158 w159] -> w138
          frame False {
          }
          frame True {
            w167 = T7[] [enum."LL", enum."HL", enum."LH", enum."HH"] items=["LL", "HL", "LH", "HH"]
            w179 = "UIdisplay" ("Process (\"\" - local)")
            n46 = for {
              tunnel: w167 -> [w187] mode=indexing
              shift-right: [w189] -> w165
              shift-left: w170 -> [w190]
              shift-right: [w184] -> w164
              shift-left: "" -> [w183]
              tunnel: [w181] -> w162
              n47 = call "set_task_detect.vi"("Action"=-1, "Test Point"=w187, "daemon reference in"=w190) -> ("error out"=w181:errorcluster, "response"=w188:string, "daemon reference out"=w189:refnum<k5>)  [unwired: 5 in, 1 out]
              n48 = Concatenate Strings(w188, ";" ("字符串")) -> (w182:string)
              n49 = Concatenate Strings(w183, w182) -> (w184:string)
            }
            n50 = call "set_calibration.vi"("error in (no error)"=w162, "values"=dbl[] [-1.0], "calibration"=T6[] ["eol_inlet_blockage"], "daemon reference in"=w165) -> ("error out"=w161:errorcluster, "response"=w160:string, "daemon reference out"=w159:refnum<k5>)  [unwired: 4 in, 1 out]
            n51 = Concatenate Strings(w164, w160) -> (w163:string)
            n52 = call "Select_Table_Vaule.vi"("Vaule"=w163, "Action"=w171, "Table"=w172) -> ("Result"=w173:bool, "vaule"=w180:string[])  [unwired: 7 in]
            n53 = Append True/False String(1:w173, 2:"FAIL" ("真字符串"), 3:"PASS" ("真字符串")) -> (0:w174:string)  [unwired: 1 in]
            n54 = Build Array (concatenate)(w180, w163, w174) -> (w178:string[])
            n55 = Flatten To XML(anything=w178) -> (xml string=w177:string)
            n56 = call "AMC Send Local Message.vi"("Process (\"\" - local)"=w179, "Message Value"=w177, "Message Name"=w179) -> ()  [unwired: 7 in, 2 out]
          }
        }
        n57 = call <vilib>:"Space Constant.vi"() -> ("String"=w150:string)
        n58 = Concatenate Strings(w147, w150, w149) -> (w151:string)
        n59 = Bundle By Name(cluster=w140, "daemon reference"=w138) -> (w139:T1)
        n60 = call "LogStatus.vi"("error in (no error)"=w142, "last message"=w153, "message"=w151) -> ("error  out"=w154:errorcluster)  [unwired: 8 in]
        n61 = case shown="错误" w142 {
          tunnel: [_ TRUE] -> w143
          tunnel: [_ "Error"] -> w144
          frame No Error {
          }
          frame Error {
          }
        }
      }
      frame "LL_Restriction" {
        w209 = "UIdisplay" ("Process (\"\" - local)")
        n62 = Unbundle By Name(w191) -> ("Table"=w198:string[][])
        n63 = call "Select_Table_Vaule Enable_Disable.vi"("Action"=w197, "Table"=w198) -> ("Enable"=w195:bool, "vaule"=w196:string[])  [unwired: 8 in]
        n64 = call "LogStatus.vi"("error in (no error)"=w221, "last message"=w220, "message"=w197) -> ("error  out"=w219:errorcluster)  [unwired: 8 in]
        n65 = case shown="真" w195 {
          tunnel: w219 -> [w224 w236]
          tunnel: [w224 w235] -> w218
          tunnel: w217 -> [w226 w234]
          tunnel: [w226 w233] -> w216
          tunnel: [w225 w232] -> w215
          tunnel: w208 -> [w225 w231]
          tunnel: ["HL_Restriction" w230] -> w202
          tunnel: w191 -> [w222 w229]
          tunnel: [w222 w228] -> w193
          tunnel: w192 -> [_ w227]
          frame False {
          }
          frame True {
            n66 = call "5.0.1_LL_Restriction.vi"("Data in"=w229, "error in (no error)"=w236, "AllControls In"=w227, 10:w231, "Message Queue out"=w234) -> ("error out"=w235:errorcluster, "Flow"=w230:string, "Data"=w232:T3, "Message Queue Out"=w233:T4, "Data out"=w228:T1)  [unwired: 2 in]
          }
        }
        n67 = Select(t="Enable" ("元素"), s=w195, f="Disable" ("元素")) -> (s? t:f=w194:string)
        n68 = Flush Queue(queue=w216) -> (queue out=w201:T4)  [unwired: 1 in, 2 out]
        n69 = Append True/False String(1:w195, 2:"FAIL" ("真字符串"), 3:"PASS" ("真字符串")) -> (0:w214:string)  [unwired: 1 in]
        n70 = Build Array (concatenate)(w196, w194, w214) -> (w212:string[])
        n71 = Flatten To XML(anything=w212) -> (xml string=w213:string)
        n72 = call "AMC Send Local Message.vi"("Process (\"\" - local)"=w209, "Message Value"=w213, "Message Name"=w209) -> ()  [unwired: 7 in, 2 out]
        n73 = Equal?(x=w202, y="Finalization_NG_unit") -> (x = y?=w205:bool)
        n74 = Equal?(x=w202, y="Error") -> (x = y?=w203:bool)
        n75 = Or(x=w205, y=w203) -> (x .or. y?=w206:bool)
      }
      frame "HL_Restriction" {
        w247 = "UIdisplay" ("Process (\"\" - local)")
        n76 = Unbundle By Name(w237) -> ("Table"=w242:string[][])
        n77 = call "Select_Table_Vaule Enable_Disable.vi"("Action"=w241, "Table"=w242) -> ("Enable"=w240:bool, "vaule"=w244:string[])  [unwired: 8 in]
        n78 = call "LogStatus.vi"("error in (no error)"=w267, "last message"=w266, "message"=w241) -> ("error  out"=w265:errorcluster)  [unwired: 8 in]
        n79 = case shown="真" w240 {
          tunnel: w265 -> [w270 w282]
          tunnel: [w270 w281] -> w264
          tunnel: w263 -> [w272 w280]
          tunnel: [w272 w279] -> w262
          tunnel: [w271 w278] -> w261
          tunnel: w260 -> [w271 w277]
          tunnel: ["LH_Restriction" w276] -> w255
          tunnel: w237 -> [w268 w275]
          tunnel: [w268 w274] -> w239
          tunnel: w238 -> [_ w273]
          frame False {
          }
          frame True {
            n80 = call "5.0.2_HL_Restriction.vi"("Data in"=w275, "error in (no error)"=w282, "AllControls In"=w273, 10:w277, "Message Queue out"=w280) -> ("error out"=w281:errorcluster, "Flow"=w276:string, "Data"=w278:T3, "Message Queue Out"=w279:T4, "Data out"=w274:T1)  [unwired: 2 in]
          }
        }
        n81 = Select(t="Enable" ("元素"), s=w240, f="Disable" ("元素")) -> (s? t:f=w243:string)
        n82 = Append True/False String(1:w240, 2:"FAIL" ("真字符串"), 3:"PASS" ("真字符串")) -> (0:w252:string)  [unwired: 1 in]
        n83 = Flush Queue(queue=w262) -> (queue out=w253:T4)  [unwired: 1 in, 2 out]
        n84 = Build Array (concatenate)(w244, w243, w252) -> (w250:string[])
        n85 = Flatten To XML(anything=w250) -> (xml string=w251:string)
        n86 = call "AMC Send Local Message.vi"("Process (\"\" - local)"=w247, "Message Value"=w251, "Message Name"=w247) -> ()  [unwired: 7 in, 2 out]
        n87 = Equal?(x=w255, y="Finalization_NG_unit") -> (x = y?=w258:bool)
        n88 = Equal?(x=w255, y="Error") -> (x = y?=w256:bool)
        n89 = Or(x=w258, y=w256) -> (x .or. y?=w254:bool)
      }
      frame "LH_Restriction" {
        w293 = "UIdisplay" ("Process (\"\" - local)")
        n90 = Unbundle By Name(w283) -> ("Table"=w288:string[][])
        n91 = call "Select_Table_Vaule Enable_Disable.vi"("Action"=w287, "Table"=w288) -> ("Enable"=w286:bool, "vaule"=w290:string[])  [unwired: 8 in]
        n92 = call "LogStatus.vi"("error in (no error)"=w313, "last message"=w312, "message"=w287) -> ("error  out"=w311:errorcluster)  [unwired: 8 in]
        n93 = case shown="真" w286 {
          tunnel: w311 -> [w316 w328]
          tunnel: [w316 w327] -> w310
          tunnel: w309 -> [w318 w326]
          tunnel: [w318 w325] -> w308
          tunnel: [w317 w324] -> w307
          tunnel: w306 -> [w317 w323]
          tunnel: ["HH_Restriction" w322] -> w300
          tunnel: [w314 w320] -> w285
          tunnel: w283 -> [w314 w321]
          tunnel: w284 -> [_ w319]
          frame False {
          }
          frame True {
            n94 = call "5.0.3_LH_Restriction.vi"("Data in"=w321, "error in (no error)"=w328, "AllControls In"=w319, 10:w323, "Message Queue out"=w326) -> ("error out"=w327:errorcluster, "Flow"=w322:string, "Data"=w324:T3, "Message Queue Out"=w325:T4, "Data out"=w320:T1)  [unwired: 2 in]
          }
        }
        n95 = Select(t="Enable" ("元素"), s=w286, f="Disable" ("元素")) -> (s? t:f=w289:string)
        n96 = Append True/False String(1:w286, 2:"FAIL" ("真字符串"), 3:"PASS" ("真字符串")) -> (0:w298:string)  [unwired: 1 in]
        n97 = Flush Queue(queue=w308) -> (queue out=w299:T4)  [unwired: 1 in, 2 out]
        n98 = Build Array (concatenate)(w290, w289, w298) -> (w296:string[])
        n99 = Flatten To XML(anything=w296) -> (xml string=w297:string)
        n100 = call "AMC Send Local Message.vi"("Process (\"\" - local)"=w293, "Message Value"=w297, "Message Name"=w293) -> ()  [unwired: 7 in, 2 out]
        n101 = Equal?(x=w300, y="Finalization_NG_unit") -> (x = y?=w304:bool)
        n102 = Equal?(x=w300, y="Error") -> (x = y?=w302:bool)
        n103 = Or(x=w304, y=w302) -> (x .or. y?=w301:bool)
      }
      frame "HH_Restriction" {
        w339 = "UIdisplay" ("Process (\"\" - local)")
        n104 = Unbundle By Name(w329) -> ("Table"=w334:string[][])
        n105 = call "Select_Table_Vaule Enable_Disable.vi"("Action"=w333, "Table"=w334) -> ("Enable"=w332:bool, "vaule"=w336:string[])  [unwired: 8 in]
        n106 = call "LogStatus.vi"("error in (no error)"=w355, "last message"=w354, "message"=w333) -> ("error  out"=w353:errorcluster)  [unwired: 8 in]
        n107 = call "5.0.4_HH_Restriction.vi"("Data in"=w329, "error in (no error)"=w353, "AllControls In"=w331, 10:w348, "Message Queue out"=w351) -> ("error out"=w352:errorcluster, "Flow"=w347:string, "Data"=w349:T3, "Message Queue Out"=w350:T4, "Data out"=w330:T1)  [unwired: 2 in]
        n108 = Flush Queue(queue=w350) -> (queue out=w345:T4)  [unwired: 1 in, 2 out]
        n109 = Select(t="Enable" ("元素"), s=w332, f="Disable" ("元素")) -> (s? t:f=w335:string)
        n110 = Append True/False String(1:w332, 2:"FAIL" ("真字符串"), 3:"PASS" ("真字符串")) -> (0:w344:string)  [unwired: 1 in]
        n111 = Build Array (concatenate)(w336, w335, w344) -> (w342:string[])
        n112 = Flatten To XML(anything=w342) -> (xml string=w343:string)
        n113 = call "AMC Send Local Message.vi"("Process (\"\" - local)"=w339, "Message Value"=w343, "Message Name"=w339) -> ()  [unwired: 7 in, 2 out]
      }
    }
    n114 = call "6-AlarmStatus.vi"("Step"=enum16{"Initial", "Write", "Read"}."Read") -> ("AlarmValue Out"=w18:bool[])  [unwired: 9 in, 1 out]
    n115 = call "Stop.vi"("Step"=enum16{"Initial", "Write", "Read"}."Read") -> ("Stop Out"=w26:bool)  [unwired: 9 in, 1 out]
    n116 = call "Exit.vi"("Step"=enum16{"Initial", "Write", "Read"}."Read" ("step")) -> ("Exit Out"=w25:bool)  [unwired: 9 in, 1 out]
    n117 = Or Array Elements(Boolean array=w18) -> (logical OR=w17:bool)
    n118 = Compound Arithmetic op=OR(w24, w26, w25, w17) -> (w23:bool)
    n119 = call "AMC Run Step.vi"("Message Queue In"=w44, "Message Name"=w32, "Message Value"=w30, "error in (no error)"=w39, "Mli/Sig"=FALSE) -> ("Message Queue Out"=w43:T4, "error out"=w38:errorcluster)  [unwired: 13 in]
  }
  "Message Queue Out" <- w6
  "error out" <- w5
  "Data" <- w10
  "Flow" <- w7
  "Data out" <- w2
